vi "Reset-image-size.vi"(8 "error in (no error)":errorcluster, 11 "PF_MV1-D1312-240 in":refnum<class "PF_MV1-D1312-240.lvclass">) -> (0 "error out":errorcluster, 1 "Image height":i32, 2 "Image width":i32, 3 "PF_MV1-D1312-240 out":refnum<class "PF_MV1-D1312-240.lvclass">)   [LabVIEW 2013, in "CameraVision.lvlib" / "PF_MV1-D1312-240.lvclass"]
uses:
  PF_MV1-D1312-240.lvclass
  Camera.lvclass/Camera.ctl
  <userlib>/Photonfocus Toolkit/_Public/SubVIs/pf_Get_Camera_Property_Int.vi
  Camera.lvclass
  <userlib>/Photonfocus Toolkit/Photonfocus_Toolkit.lvlib
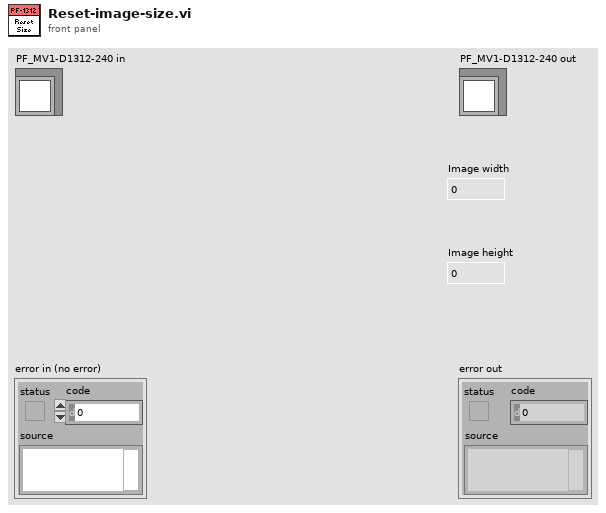
[diagram p1: front panel]
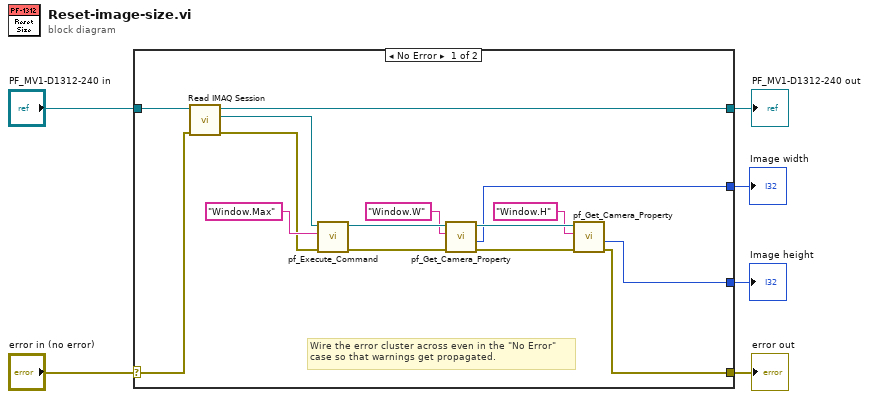
[diagram p0: block diagram]
diagram:
  n1 = case shown="No Error" "error in (no error)" {
    selector: "error in (no error)" -> [w19 w23]
    tunnel: [w10 w23] -> w5
    tunnel: [w20 w22] -> w3
    tunnel: "PF_MV1-D1312-240 in" -> [w21 w22]
    tunnel: [w9 _] -> w2
    tunnel: [w7 _] -> w1
    frame No Error {
      # "Wire the error cluster across even in the \"No Error\"\ncase so that warnings get propagated."
      n2 = call "Read IMAQ Session.vi"("error in (no error)"=w19, "Camera in"=w21) -> ("error out"=w16:errorcluster, "IMAQ Session"=w17:refnum<k11>, "Camera out"=w20:refnum<class "PF_MV1-D1312-240.lvclass">)  [unwired: 7 in]
      n3 = call <userlib>:"pf_Execute_Command.vi"("error in (no error)"=w16, "Command"="Window.Max" ("Property Name"), "IMAQ Session in"=w17) -> ("error out"=w14:errorcluster, "IMAQ Session out"=w15:refnum<k11>)  [unwired: 7 in]
      n4 = call-poly <userlib>:"pf_Get_Camera_Property.vi"("error in (no error)"=w14, "Property Name"="Window.W", "IMAQ Session in"=w15) -> ("error out"=w12:errorcluster, "Property Value"=w9:i32, "IMAQ Session out"=w11:refnum<k11>)  [unwired: 5 in, 1 out]
      n5 = call-poly <userlib>:"pf_Get_Camera_Property.vi"("error in (no error)"=w12, "Property Name"="Window.H", "IMAQ Session in"=w11) -> ("error out"=w10:errorcluster, "Property Value"=w7:i32)  [unwired: 5 in, 2 out]
    }
    frame Error {
    }
  }
  "error out" <- w5
  "PF_MV1-D1312-240 out" <- w3
  "Image width" <- w2
  "Image height" <- w1
